vi "MenuHandler.vi"(5 "tree control":refnum<vi>, 7 "main queue":T1, 8 "error in":errorcluster, 9 "parameters":variant, 10 "menu string":string, 11 "CEF_Node in":refnum<class "CEF_Node.lvclass">) -> (0 "error out":errorcluster, 1 "refresh tree?":bool, 2 "Unhandled":bool, 3 "CEF_Node out":refnum<class "CEF_Node.lvclass">)   [LabVIEW 2025, in "CEF.lvlib" / "CEF_Node.lvclass"]
doc: "Copyright 2017 National Instruments Corporation\n\nLicensed under the Apache License, Version 2.0 (the \"License\"); you may not use this file except in compliance with the License. You may obtain a copy of the License at http://www.apache.org/licenses/LICENSE-2.0\nUnless required by applicable law or agreed to in writing, software distributed under the License is distributed on an \"AS IS\" BASIS, WITHOUT WARRANTIES OR CONDITIONS OF ANY KIND, either express or implied. See the License for the specific language governing permissions and limitations under the License."
uses:
  CEF_Node.lvclass
  mainQref.ctl
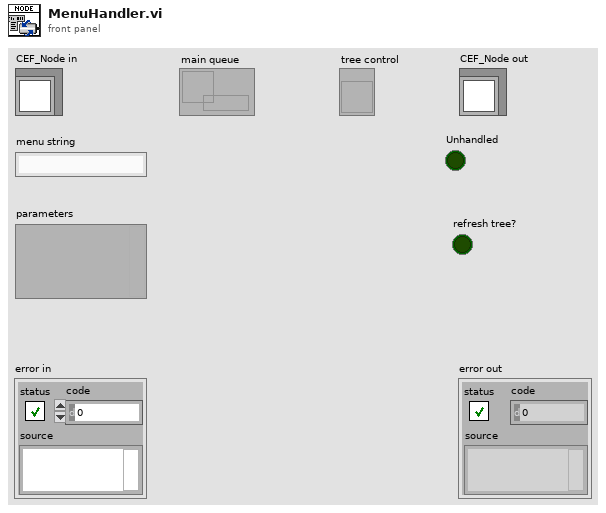
[diagram p1: front panel]
types:
  T1 = typedef "CEF.lvlib/CEF_Node.lvclass/mainQref.ctl" = refnum<queue>
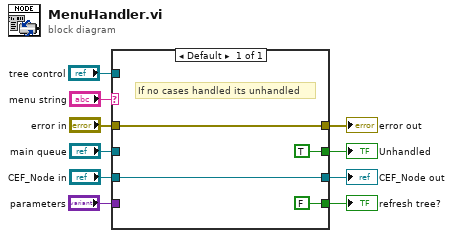
[diagram p0: block diagram]
diagram:
  n1 = case shown="Default" "menu string" {
    tunnel: [TRUE ("Unhandled")] -> w9
    tunnel: "parameters" -> [_]
    tunnel: "tree control" -> [_]
    tunnel: "main queue" -> [_]
    tunnel: "CEF_Node in" -> [w13]
    tunnel: [w13] -> w4
    tunnel: [w12] -> w2
    tunnel: "error in" -> [w12]
    tunnel: [FALSE] -> w1
    frame Default {
      # "If no cases handled its unhandled"
    }
  }
  "error out" <- w2
  "CEF_Node out" <- w4
  "Unhandled" <- w9
  "refresh tree?" <- w1
